vi "HandleMenu.vi"(7 "message queue":T1, 8 "error in":errorcluster, 9 "Item Path":string, 10 "ItemTag":string, 11 "NISE_CEF_Repository in":refnum<class "NISE_CEF_Repository.lvclass">) -> (0 "error out":errorcluster, 2 "handled?":bool, 3 "NISE_CEF_Repository out":refnum<class "NISE_CEF_Repository.lvclass">)   [LabVIEW 2013, in "NISE_CEF_Repository.lvclass"]
uses:
  NISE_CEF_Repository.lvclass
  <vilib>/NI/AMC/Message Queue.ctl
  <vilib>/NI/AMC/Message.ctl
  <vilib>/NI/Tools/Keyed Array/KeyedArray.ctl
  <vilib>/NI/AMC/AMC.lvlib
  <vilib>/NI/Tools/Keyed Array/Tools_KeyedArray.lvlib
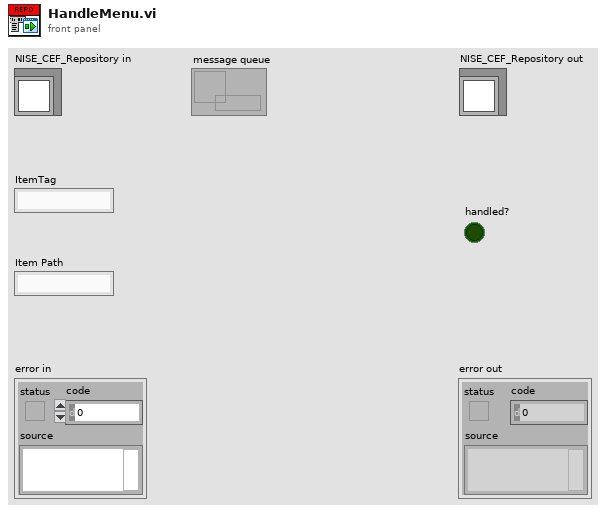
[diagram p1: front panel]
types:
  T1 = typedef "AMC.lvlib/Message Queue.ctl" = refnum<queue>
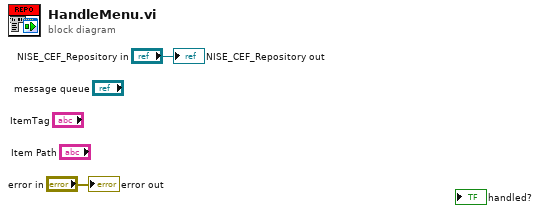
[diagram p0: block diagram]
diagram:
  "error out" <- "error in"
  "NISE_CEF_Repository out" <- "NISE_CEF_Repository in"
